vi "Returning Values By Reference String.vi"(8 "error in (no error)":errorcluster, 10 "newString":string, 11 "str":string) -> (0 "error out":errorcluster, 2 "newString out":string, 3 "str out":string)   [LabVIEW 2009, in "LabVIEWWrapper_PassingDataSampleDLL.lvlib"]
doc: "void ReturningValuesByReference_String (char *str, char **newString);"
uses:
  LabVIEWWrapper_PassingDataSampleDLL.lvlib
  PassingDataSampleDLL.dll
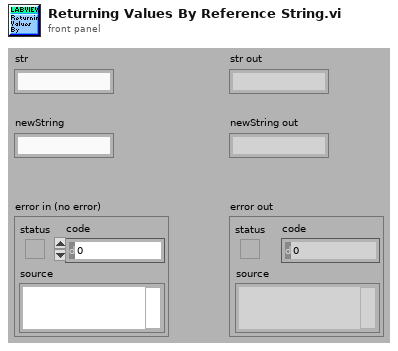
[diagram p1: front panel]
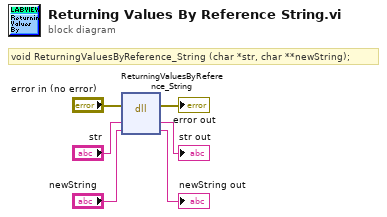
[diagram p0: block diagram]
diagram:
  # "void ReturningValuesByReference_String (char *str, char **newString);"
  n1 = dll-call lib="C:/My Dropbox/Systems Engineering Application/SDK/C Integration/LabVIEWWrapper/PassingDataSampleDLL.*" fn="ReturningValuesByReference_String"(error in="error in (no error)", "str"="str", "newString"="newString") -> (error out=→"error out":errorcluster, "str"=→"str out":string, "newString"=→"newString out":string)  [unwired: 3 in, 1 out]
